vi "WriteResults.vi"(5 "EVMHignLimit":i32 format="%.1f", 6 "Mask":dbl, 7 "EVM":dbl format="%#.4f", 8 "error in (no error)":errorcluster, 9 "Power":dbl, 10 "FreqError":dbl format="%#_4f", 11 "refnum out":refnum<file>) -> (0 "error out":errorcluster, 3 "refnum out 2":refnum<file>)   [LabVIEW 2012]
panel:
  out "resulting string":string
  out "concatenated string":string
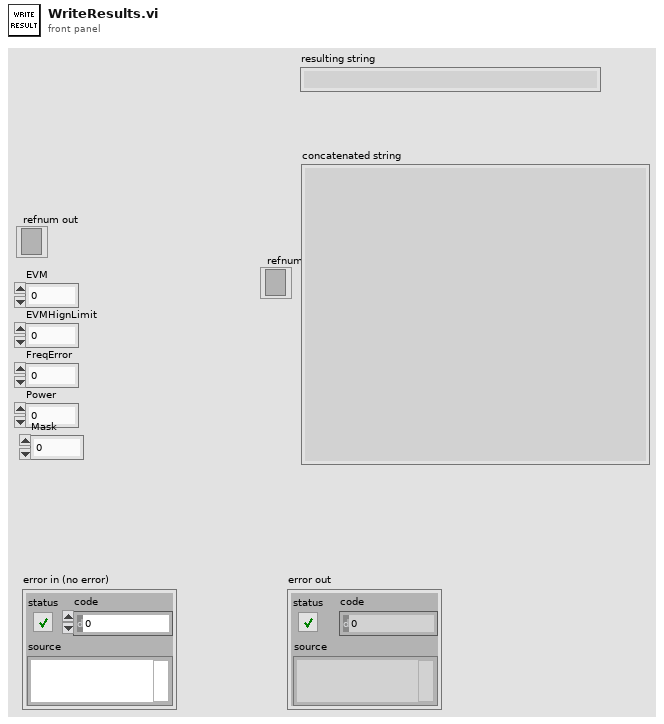
[diagram p1: front panel]
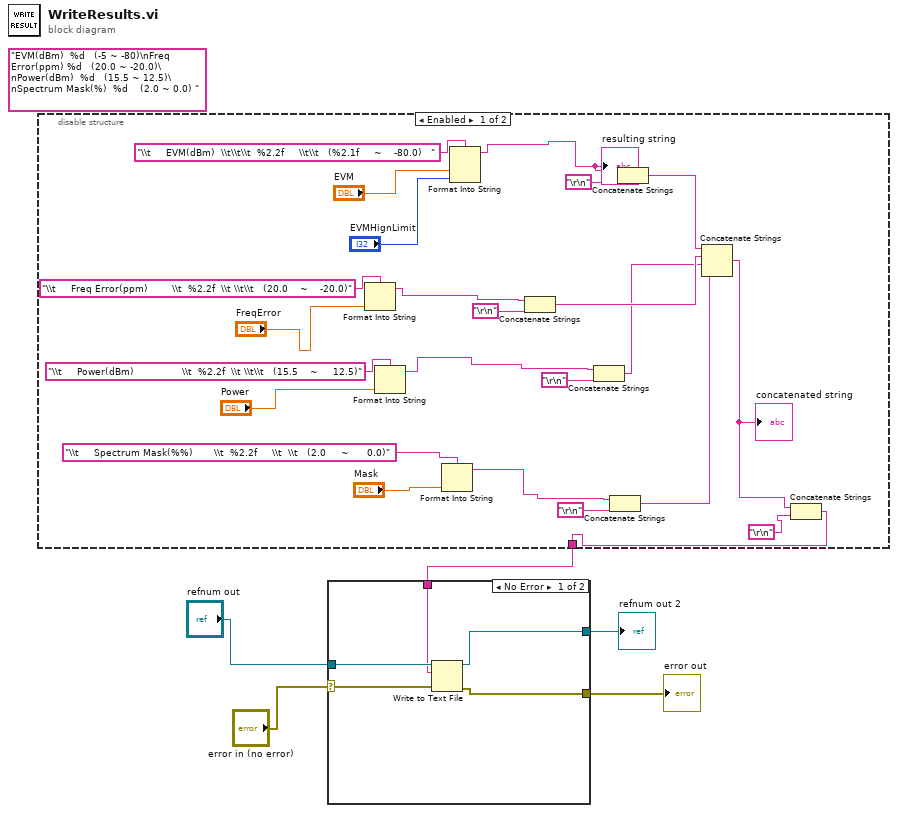
[diagram p0: block diagram]
diagram:
  (unwired) "EVM(dBm)  %d   (-5 ~ -80)\nFreq Error(ppm) %d   (20.0 ~ -20.0)\nPower(dBm)  %d   (15.5 ~ 12.5)\nSpectrum Mask(%)  %d    (2.0 ~ 0.0) " ("format string")
  n1 = disable-structure shown="Enabled" {
    disable-tunnel: [w6 _] -> w2
    frame Enabled {
      n2 = Format Into String(format string="\\t     Freq Error(ppm)        \\t  %2.2f  \\t \\t\\t   (20.0    ~    -20.0)" ("initial string"), "FreqError") -> (resulting string=w11:string)  [unwired: 2 in, 1 out]
      n3 = Format Into String(format string="\\t     Power(dBm)                \\t  %2.2f  \\t \\t\\t   (15.5    ~     12.5)" ("initial string"), "Power") -> (resulting string=w10:string)  [unwired: 2 in, 1 out]
      n4 = Format Into String(format string="\\t     Spectrum Mask(%%)       \\t  %2.2f     \\t  \\t   (2.0     ~      0.0)" ("initial string"), "Mask") -> (resulting string=w9:string)  [unwired: 2 in, 1 out]
      n5 = Format Into String(format string="\\t     EVM(dBm)  \\t\\t\\t  %2.2f     \\t\\t   (%2.1f     ~    -80.0)   " ("initial string"), "EVM", "EVMHignLimit") -> (resulting string=w12:string)  [unwired: 2 in, 1 out]
      "resulting string" <- w12
      n6 = Concatenate Strings(w11, "\r\n") -> (w20:string)
      n7 = Concatenate Strings(w10, "\r\n") -> (w19:string)
      n8 = Concatenate Strings(w9, "\r\n") -> (w18:string)
      n9 = Concatenate Strings(w12, "\r\n") -> (w21:string)
      n10 = Concatenate Strings(w21, w20, w19, w18) -> (w7:string)
      "concatenated string" <- w7
      n11 = Concatenate Strings(w7, "\r\n") -> (w6:string)
    }
    frame Disabled {
    }
  }
  n12 = case shown="No Error" "error in (no error)" {
    selector: "error in (no error)" -> [w33 w35]
    tunnel: [w32 w35] -> w4
    tunnel: "refnum out" -> [w34 _]
    tunnel: w2 -> [w31 _]
    tunnel: [w30 _] -> w1
    frame No Error {
      n13 = Write to Text File(file (use dialog)=w34, text=w31, error in=w33) -> (refnum out=w30:refnum<file>, error out=w32:errorcluster)  [unwired: 1 in, 1 out]
    }
    frame Error {
    }
  }
  "error out" <- w4
  "refnum out 2" <- w1
